vi "CALCU_VI.vi"() -> ()   [LabVIEW 2021]
doc: "This VI calculates the value for the following operations with operand as M and N.\na. Factorial of M+N\nb. Sum of factorials of first M natural numbers\nc. Sum of factorials of first N whole numbers\nd. Greater of M and N"
panel:
  out "C":i64
  in  "Stop":bool
  in  "Operations":T1(ring)
  in  "N":i64
  in  "M":i64
  # "CALCULATE THE OUTPUT 'C'"
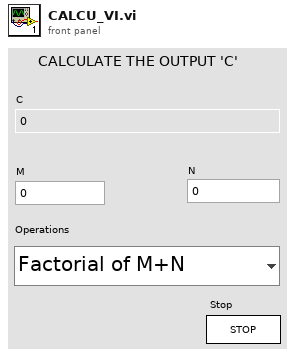
[diagram p1: front panel]
types:
  T1 = enum16{"Factorial of M+N", "Sum of factorials of first M natural numbers", "Sum of factorials of first N whole number", "Greater of M and N"}
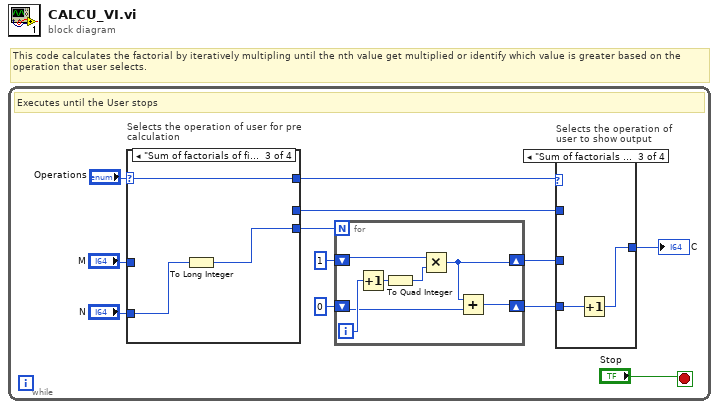
[diagram p0: block diagram]
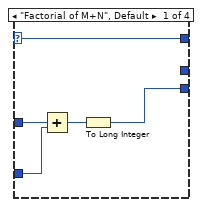
[diagram p5: hidden frame]
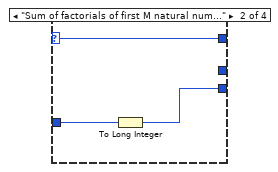
[diagram p6: hidden frame]
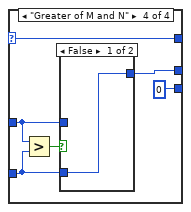
[diagram p7: hidden frame]
diagram:
  # "This code calculates the factorial by iteratively multipling until the nth value get multiplied or identify which value is greater based on the operation that user selects."
  n1 = while {
    stop <- "Stop" stop-if-true
    # "Executes until the User stops"
    n2 = case "Selects the operation of user for pre calculation" shown="\"Sum of factorials of first N whole number\"" "Operations" {
      selector: "Operations" -> [w25 w30 w33 w38]
      tunnel: "M" -> [w29 w32 _ w40]
      tunnel: "N" -> [w28 _ w35 w39]
      tunnel: [w26 w31 w34 0] -> w8
      tunnel: [w25 w30 w33 w38] -> w5
      tunnel: [_ _ _ w36] -> w1
      frame "Factorial of M+N", Default {
        n3 = Add(x=w29, y=w28) -> (x+y=w27:i64)
        n4 = To Long Integer(number=w27) -> (32bit integer=w26:i32)
      }
      frame "Sum of factorials of first M natural numbers" {
        n5 = To Long Integer(number=w32) -> (32bit integer=w31:i32)
      }
      frame "Sum of factorials of first N whole number" {
        n6 = To Long Integer(number=w35) -> (32bit integer=w34:i32)
      }
      frame "Greater of M and N" {
        # "Selects the command for execution"
        n7 = Greater?(x=w40, y=w39) -> (0:w41:bool)
        n8 = case shown="False" w41 {
          tunnel: w40 -> [_ w43]
          tunnel: w39 -> [w42 _]
          tunnel: [w42 w43] -> w36
          frame False {
          }
          frame True {
          }
        }
      }
    }
    n9 = for {
      N: w8 -> [_]
      shift-right: [w20] -> w4
      shift-left: i64 1 -> [w24]
      shift-right: [w19] -> w2
      shift-left: i64 0 -> [w18]
      i -> [w23]
      n10 = Increment(x=w23) -> (x+1=w22:i32)
      n11 = To Quad Integer(1:w22) -> (0:w21:i64)
      n12 = Multiply(x=w24, y=w21) -> (x*y=w20:i64)
      n13 = Add(x=w20, y=w18) -> (x+y=w19:i64)
    }
    n14 = case "Selects the operation of user to show output" shown="\"Sum of factorials of first N whole number\"" w5 {
      tunnel: w4 -> [w13 _ _ _]
      tunnel: [w13 w14 w15 w17] -> w3
      tunnel: w2 -> [_ w14 w16 _]
      tunnel: w1 -> [_ _ _ w17]
      frame "Factorial of M+N", Default {
      }
      frame "Sum of factorials of first M natural numbers" {
      }
      frame "Sum of factorials of first N whole number" {
        n15 = Increment(x=w16) -> (x+1=w15:i64)
      }
      frame "Greater of M and N" {
        # "Selects the command for display output"
      }
    }
    "C" <- w3
  }
